vi "AdsStateChanged Event Callback.vi"(4 "User Parameter":refnum<user-event>, 5 "Event Data":cluster{"sender":refnum<k24>, "e":refnum<k24>}, 6 "Control Ref":refnum<k24>, 7 "Event Common Data":T1) -> ()   [LabVIEW 2018, in "TwinCAT ADS.lvclass"]
uses:
  TwinCAT ADS.lvclass
  TwinCAT.Ads
  Controls/State Information.ctl
  <vilib>/event_ctls.llb/usereventprio.ctl
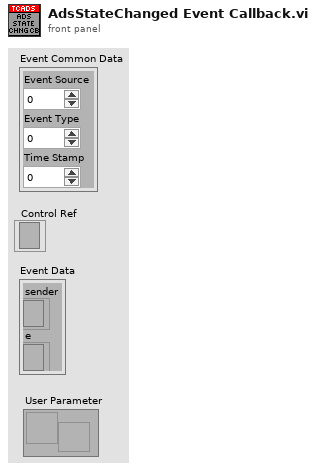
[diagram p1: front panel]
types:
  T1 = cluster{"Event Source":i32, "Event Type":u32, "Time Stamp":u32}
  T2 = typedef "usereventprio.ctl" = enum32{"high priority", "normal priority"}
  T3 = typedef "TwinCAT ADS.lvclass/State Information.ctl" = cluster{"ADS State":enum16{"Invalid", "Idle", "Reset", "Init", "Start", "Run", "Stop", "SaveConfig", "LoadConfig", "PowerFailure", "PowerGood", "Error", "Shutdown", "Suspend", "Resume", "Config", "Reconfig", "Stopping, Maxstates", "Incompatible", "Exception"}, "Device State":i16}
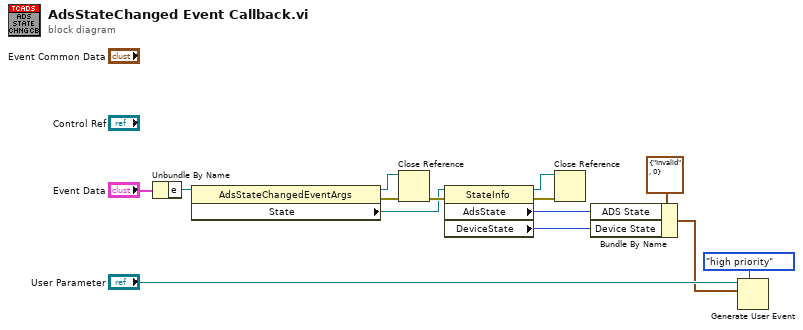
[diagram p0: block diagram]
diagram:
  n1 = Unbundle By Name("Event Data") -> ("e"=w13:refnum<k24>)
  n2 = property class="AdsStateChangedEventArgs"(reference=w13) -> (reference out=w11:refnum<k24>, error out=w12:errorcluster, "State"=w9:refnum<k24>)  [unwired: 1 in]
  n3 = Close Reference(reference=w11, error in (no error)=w12) -> (error out=w10:errorcluster)
  n4 = property class="StateInfo"(reference=w9, error in=w10) -> (reference out=w7:refnum<k24>, error out=w8:errorcluster, "AdsState"=w4:i16, "DeviceState"=w3:i16)
  n5 = Close Reference(reference=w7, error in (no error)=w8) -> ()  [unwired: 1 out]
  n6 = Bundle By Name(cluster=T3 {"ADS State"=enum."Invalid", "Device State"=0} ("State Information"), "ADS State"=w4, "Device State"=w3) -> (w2:T3)
  n7 = Generate User Event(priority (normal)=usereventprio."high priority", user event="User Parameter", event data cluster=w2) -> ()  [unwired: 1 in, 2 out]
